vi "Do.vi"(8 "error in":errorcluster, 10 "Actor in":refnum<class "Actor.lvclass">, 11 "Set Vrange MSG":refnum<class "Set Vrange MSG.lvclass">) -> (0 "error out":errorcluster, 2 "Actor out":refnum<class "Actor.lvclass">)   [LabVIEW 2014, in "ePAS Library.lvlib" / "Set Vrange MSG.lvclass"]
doc: "(<B>Filename</B>: Actor Framework.lvlib:Message.lvclass:Do.vi)\n\nDefines what a message does when it is received by an actor. Generally, a message instructs an actor to invoke one of its methods. By default, this method does nothing. A child class must override it to define behavior. Create a child class by using the Actor Framework Message Maker dialog box."
uses:
  Set Vrange MSG.lvclass
  <vilib>/ActorFramework/Actor/Actor.lvclass
  Set Vrange MSG.lvclass/Set Vrange MSG.ctl
  Instr Actor.lvclass
  PAS/Commands/Change Laser Vrange/Change Laser Vrange.lvclass
  PAS/Commands/Change Laser Vrange/Change Laser Vrange.lvclass/Change Laser Vrange.ctl
  Controller/Messages/Update CVT/Update CVT Data.lvclass
  Controller/Messages/Update CVT/Update CVT Data.lvclass/Update CVT Data.ctl
  Controller/Messages/Update CVT/Write tag.vi
  Controller/Messages/Update CVT/Write Data.vi
  Controller/Messages/Update CVT/Write Group.vi
  PAS/Commands/Change Laser Vrange/Write Vrange.vi
  reusable/Command/Command.lvclass
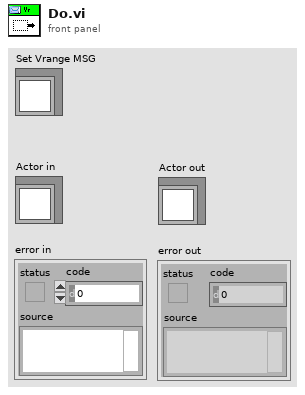
[diagram p1: front panel]
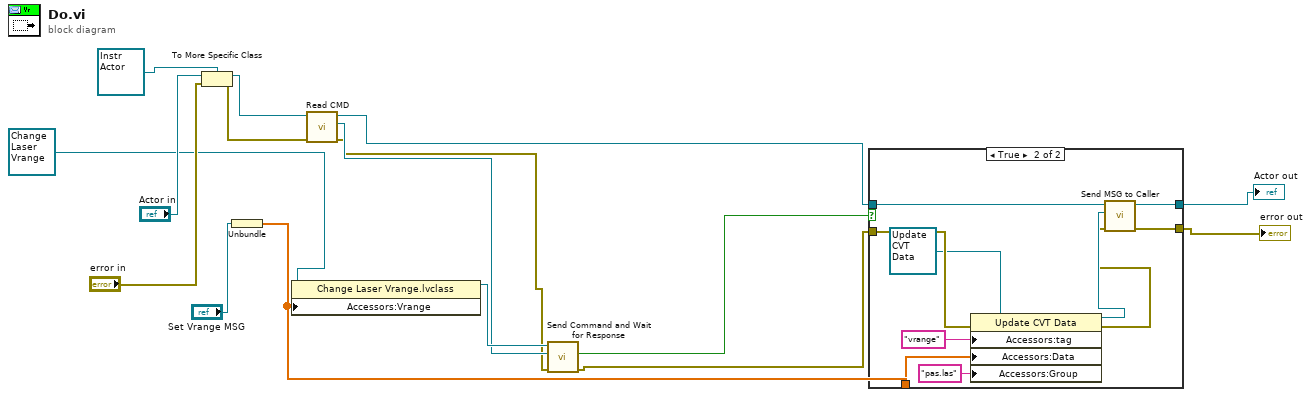
[diagram p0: block diagram]
diagram:
  n1 = To More Specific Class(target class=refnum<class "Instr Actor.lvclass"> refnum ("Instrument Lib:Instr"), reference="Actor in", error in="error in") -> (specific class reference=w14:refnum<class "Instr Actor.lvclass">, error out=w13:errorcluster)
  n2 = Unbundle("Set Vrange MSG") -> (w3:sgl[])
  n3 = property class="Change Laser Vrange.lvclass"(reference=refnum<class "Change Laser Vrange.lvclass"> refnum ("Change Laser Vrange.lvclass"), "Accessors:Vrange"=w3) -> (reference out=w9:refnum<class "Change Laser Vrange.lvclass">)  [unwired: 1 in, 1 out]
  n4 = call "Read CMD.vi"("error in (no error)"=w13, "Instr Actor in"=w14) -> ("error out"=w7:errorcluster, "CMD"=w8:refnum<queue>, "Instr Actor out"=w5:refnum<class "Instr Actor.lvclass">)  [unwired: 7 in]
  n5 = call "Send Command and Wait for Response.vi"("error in"=w7, "cmd queue"=w8, "CMD in"=w9) -> ("error out"=w4:errorcluster, "cmd good?"=w6:bool)  [unwired: 6 in, 1 out]
  n6 = case shown="True" w6 {
    tunnel: w3 -> [_ w24]
    tunnel: w5 -> [w18 w28]
    tunnel: [w18 w27] -> w1
    tunnel: w4 -> [w17 w22]
    tunnel: [w17 w26] -> w2
    frame False {
    }
    frame True {
      n7 = property class="Update CVT Data"(reference=refnum<class "Update CVT Data.lvclass"> refnum ("Controller.lvlib:Update CVT Data"), error in=w22, "Accessors:tag"="vrange" ("Key"), "Accessors:Data"=w24, "Accessors:Group"="pas.las" ("Group")) -> (reference out=w23:refnum<class "Update CVT Data.lvclass">, error out=w21:errorcluster)
      n8 = call "Send MSG to Caller.vi"("error in"=w21, "Message"=w23, "Instr in"=w28) -> ("error out"=w26:errorcluster, "Instr out"=w27:refnum<class "Instr Actor.lvclass">)  [unwired: 7 in]
    }
  }
  "error out" <- w2
  "Actor out" <- w1
